vi "Initialize camera and buffer.vi"(8 "Buffer size":i32, 9 "Image Name":string="Frame ", 11 "Session In":T1="cam0") -> (0 "error out":errorcluster, 2 "Images Out":T2[](array[typedef]), 3 "Session Out":T1)   [LabVIEW 2018]
uses:
  <vilib>/userdefined/High Color/IMAQdx.ctl
  <vilib>/vision/Image Controls.llb/IMAQ Image.ctl
  <vilib>/vision/driver/IMAQdx.llb/IMAQdx Acquisition Mode.ctl
  <vilib>/vision/driver/NI_Vision_Acquisition_Software.lvlib
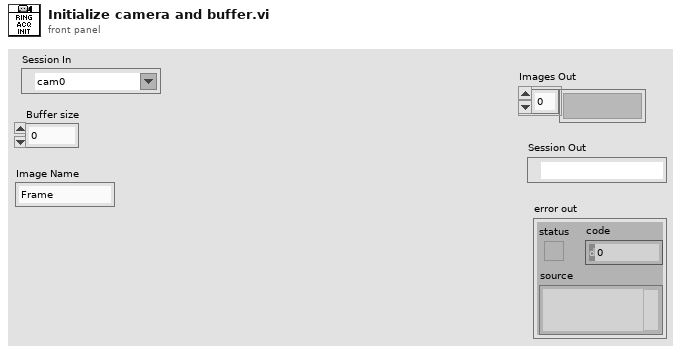
[diagram p1: front panel]
types:
  T1 = typedef "IMAQdx.ctl" = refnum<k21>
  T2 = typedef "IMAQ Image.ctl" = refnum<image>
  T3 = typedef "NI_Vision_Acquisition_Software.lvlib/IMAQdx Acquisition Mode.ctl" = enum32{"One Shot", "Continuous"}
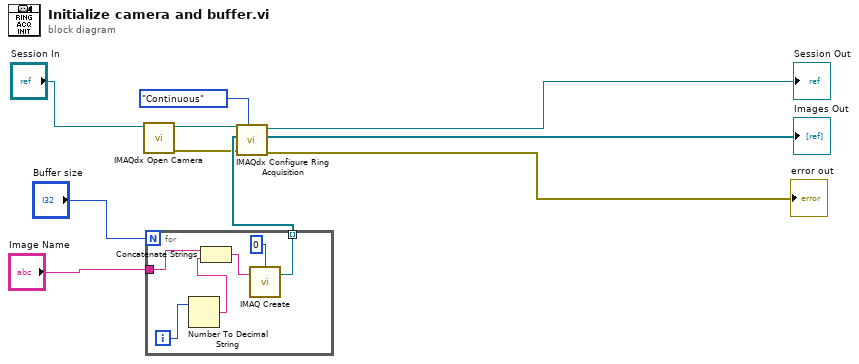
[diagram p0: block diagram]
diagram:
  n1 = call <vilib>:"IMAQdx Open Camera.vi"("Session In"="Session In") -> ("error out"=w2:errorcluster, "Session Out"=w9:T1)  [unwired: 9 in]
  n2 = for {
    N: "Buffer size" -> [_]
    tunnel: "Image Name" -> [w16]
    tunnel: [w12] -> w6 mode=indexing
    i -> [w15]
    n3 = Number To Decimal String(number=w15) -> (decimal integer string=w14:string)  [unwired: 1 in]
    n4 = Concatenate Strings(w16, w14) -> (w13:string)
    n5 = call "IMAQ Create"("Border Size"=0, "Image Name"=w13) -> ("New Image"=w12:T2)  [unwired: 3 in, 1 out]
  }
  n6 = call <vilib>:"IMAQdx Configure Ring Acquisition.vi"("Mode"=IMAQdx_Acquisition_Mode."Continuous", "error in"=w2, "Images"=w6, "Session In"=w9) -> ("error out"=→"error out":errorcluster, "Images Out"=→"Images Out":T2[], "Session Out"=→"Session Out":T1)  [unwired: 5 in]
